vi "Reset.vi"(8 "error in":errorcluster) -> (0 "error out":errorcluster)   [LabVIEW 2012]
uses:
  <vilib>/Rock Robotics/WPI/Solenoid/WPI_SolenoidValue.ctl
  <vilib>/Rock Robotics/WPI/Solenoid/WPI_SolenoidSetEnum.vi
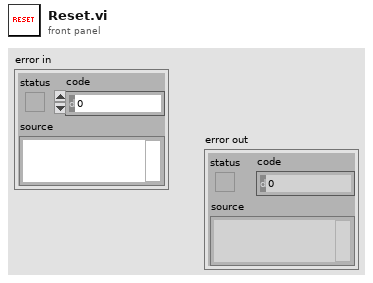
[diagram p1: front panel]
types:
  T1 = typedef "WPI_SolenoidValue.ctl" = enum16{"Off", "On", "Forward", "Reverse"}
  T2 = typedef "WPI_SolenoidDevRef.ctl" = cluster{"DevStatus":errorcluster, "Solenoid Module":T3, "Forward Solenoid Channel":T4, "Reverse Solenoid Channel":T4}
  T3 = typedef "FPGA_TypedefSolenoidModule.ctl" = enum16{"Solenoid Module 1", "Solenoid Module 2"}
  T4 = typedef "WPI_SolenoidChannel.ctl" = enum8{"Solenoid 1", "Solenoid 2", "Solenoid 3", "Solenoid 4", "Solenoid 5", "Solenoid 6", "Solenoid 7", "Solenoid 8", "Invalid"}
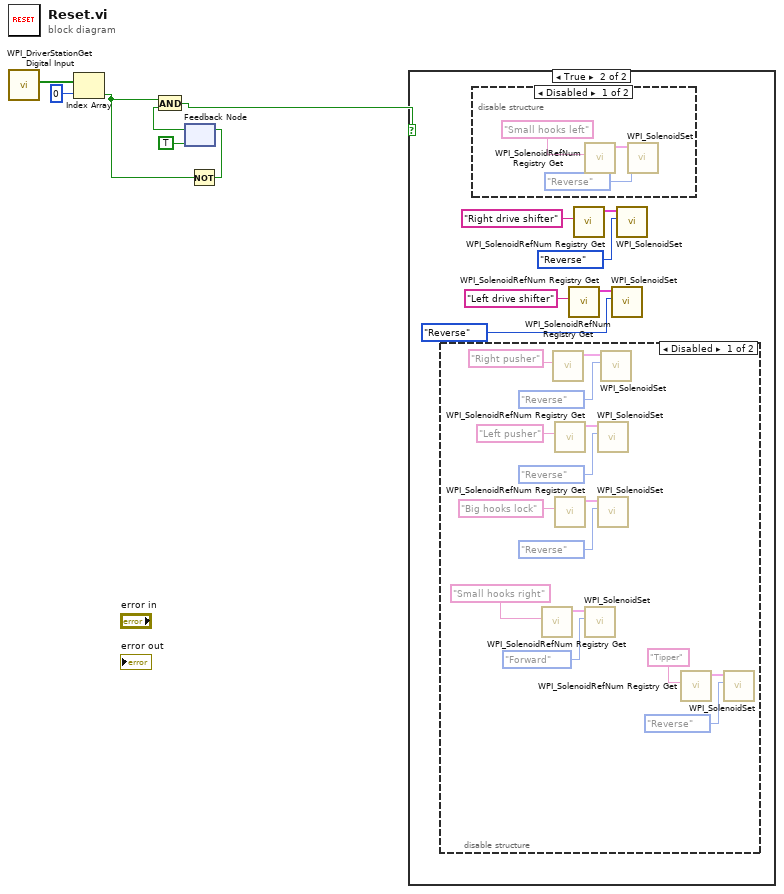
[diagram p0: block diagram]
diagram:
  n1 = call <vilib>:"WPI_DriverStationGet Digital Input.vi"() -> ("Driver Station Digital Input (1-8)"=w6:bool[])  [unwired: 11 in]
  n2 = Index Array(array=w6, index=0) -> (element=w1:bool)
  n3 = feedback #1(TRUE) -> (w2:bool)
  n4 = And(x=w1, y=w2) -> (x .and. y?=w4:bool)
  n5 = Not(x=w1) -> (.not. x?=w3:bool)
  n6 = feedback-in #1(w3) -> ()
  n7 = case shown="True" w4 {
    frame False {
    }
    frame True {
      n8 = disable-structure shown="Disabled" {
        frame Disabled {
          n9 = call <vilib>:"WPI_SolenoidRefNum Registry Get.vi"("refnum name"="Small hooks right") -> ("SolenoidDevRef"=w22:T2)  [unwired: 9 in, 1 out]
          n10 = call <vilib>:"WPI_SolenoidRefNum Registry Get.vi"("refnum name"="Right pusher") -> ("SolenoidDevRef"=w30:T2)  [unwired: 9 in, 1 out]
          n11 = call <vilib>:"WPI_SolenoidRefNum Registry Get.vi"("refnum name"="Left pusher") -> ("SolenoidDevRef"=w27:T2)  [unwired: 9 in, 1 out]
          n12 = call <vilib>:"WPI_SolenoidRefNum Registry Get.vi"("refnum name"="Big hooks lock") -> ("SolenoidDevRef"=w24:T2)  [unwired: 9 in, 1 out]
          n13 = call-poly <vilib>:"WPI_SolenoidSet.vi"("Value"=WPI_SolenoidValue."Forward", "SolenoidDevRef"=w22) -> ()  [unwired: 8 in, 2 out]
          n14 = call-poly <vilib>:"WPI_SolenoidSet.vi"("Value"=WPI_SolenoidValue."Reverse", "SolenoidDevRef"=w27) -> ()  [unwired: 8 in, 2 out]
          n15 = call-poly <vilib>:"WPI_SolenoidSet.vi"("Value"=WPI_SolenoidValue."Reverse", "SolenoidDevRef"=w24) -> ()  [unwired: 8 in, 2 out]
          n16 = call-poly <vilib>:"WPI_SolenoidSet.vi"("Value"=WPI_SolenoidValue."Reverse", "SolenoidDevRef"=w30) -> ()  [unwired: 8 in, 2 out]
          n17 = call <vilib>:"WPI_SolenoidRefNum Registry Get.vi"("refnum name"="Tipper") -> ("SolenoidDevRef"=w19:T2)  [unwired: 9 in, 1 out]
          n18 = call-poly <vilib>:"WPI_SolenoidSet.vi"("Value"=WPI_SolenoidValue."Reverse", "SolenoidDevRef"=w19) -> ()  [unwired: 8 in, 2 out]
        }
        frame Enabled {
        }
      }
      n19 = disable-structure shown="Disabled" {
        frame Disabled {
          n20 = call <vilib>:"WPI_SolenoidRefNum Registry Get.vi"("refnum name"="Small hooks left") -> ("SolenoidDevRef"=w16:T2)  [unwired: 9 in, 1 out]
          n21 = call-poly <vilib>:"WPI_SolenoidSet.vi"("Value"=WPI_SolenoidValue."Reverse", "SolenoidDevRef"=w16) -> ()  [unwired: 8 in, 2 out]
        }
        frame Enabled {
        }
      }
      n22 = call <vilib>:"WPI_SolenoidRefNum Registry Get.vi"("refnum name"="Left drive shifter") -> ("SolenoidDevRef"=w9:T2)  [unwired: 9 in, 1 out]
      n23 = call <vilib>:"WPI_SolenoidRefNum Registry Get.vi"("refnum name"="Right drive shifter") -> ("SolenoidDevRef"=w12:T2)  [unwired: 9 in, 1 out]
      n24 = call-poly <vilib>:"WPI_SolenoidSet.vi"("Value"=WPI_SolenoidValue."Reverse", "SolenoidDevRef"=w9) -> ()  [unwired: 8 in, 2 out]
      n25 = call-poly <vilib>:"WPI_SolenoidSet.vi"("Value"=WPI_SolenoidValue."Reverse", "SolenoidDevRef"=w12) -> ()  [unwired: 8 in, 2 out]
    }
  }
